vi "Controller Orbit Correction Algorithm.vi"(0 "FOFB Variables":T1, 1 "Corrector Kick Vector in":dbl[](array[numeric]), 2 "Beam Position Vector":dbl[](array[numeric]), 5 "error in (no error)":errorcluster, 9 "Reset?":bool) -> (14 "Good value?":bool=TRUE, 15 "Corrector Kick Vector out":dbl[](array[numeric]), 19 "error out":errorcluster)   [LabVIEW 2011, in "Controller VIs.lvlib"]
doc: "Computes the correction algorithm to the selected BPM readings and returns the calculated corrector kick vector to be applied to the FOFB actuators."
uses:
  Controller VIs.lvlib
  Types Definitions/Type FOFB Variables.ctl
  Common VIs.lvlib
  Type Definitions.lvlib
panel:
  in  "Maximum allowed disturbance (mm) (1.5)":dbl=1.5 format="%#_6f"
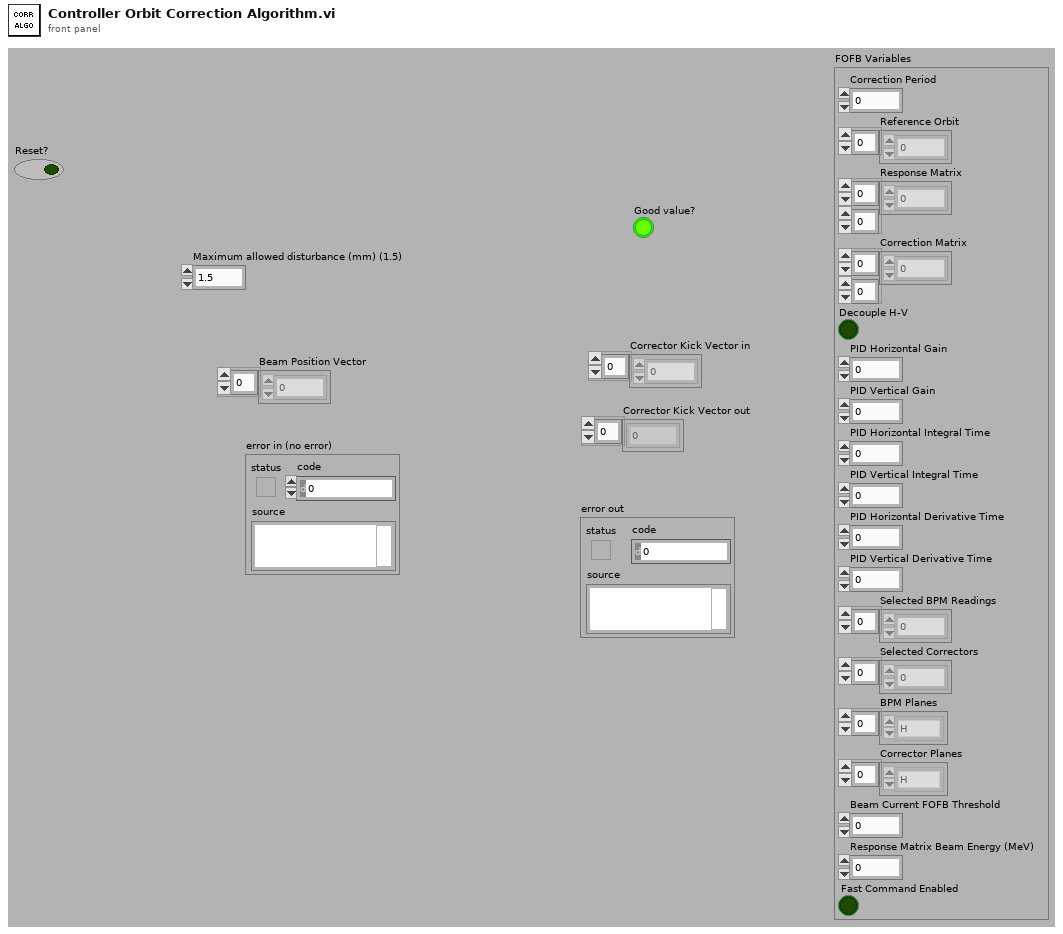
[diagram p1: front panel]
types:
  T1 = typedef "Type Definitions.lvlib/Type FOFB Variables.ctl" = cluster{"Correction Period":u32, "Reference Orbit":dbl[], "Response Matrix":dbl[][], "Correction Matrix":dbl[][], "Decouple H-V":bool, "PID Horizontal Gain":dbl, "PID Vertical Gain":dbl, "PID Horizontal Integral Time":dbl, "PID Vertical Integral Time":dbl, "PID Horizontal Derivative Time":dbl, "PID Vertical Derivative Time":dbl, "Selected BPM Readings":u32[], "Selected Correctors":u32[], "BPM Planes":enum8{"H", "V"}[], "Corrector Planes":enum8{"H", "V"}[], "Beam Current FOFB Threshold":dbl, "Response Matrix Beam Energy (MeV)":dbl, "Fast Command Enabled":bool}
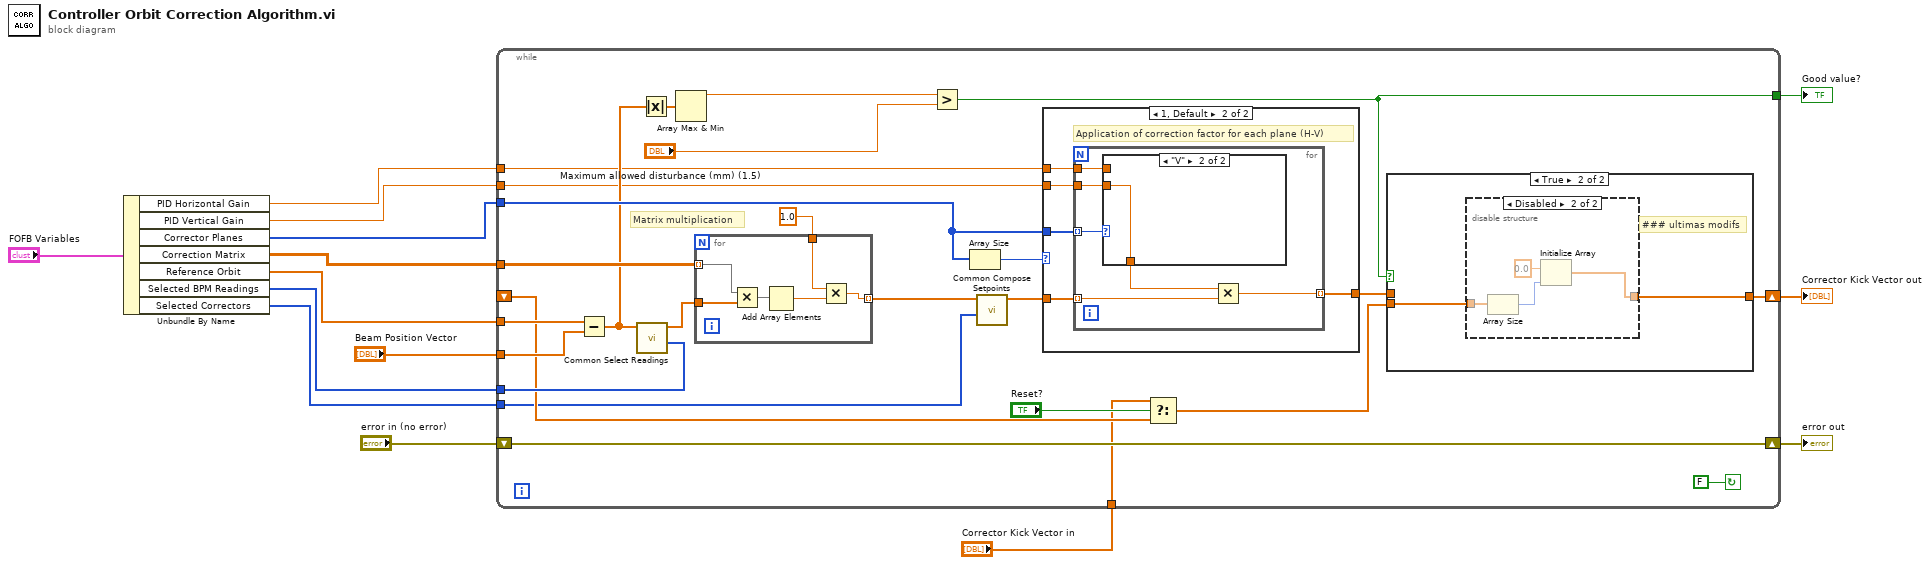
[diagram p0: block diagram]
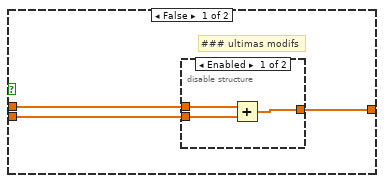
[diagram p2: hidden frame]
diagram:
  n1 = Unbundle By Name("FOFB Variables") -> ("PID Horizontal Gain"=w1:dbl, "PID Vertical Gain"=w2:dbl, "Corrector Planes"=w3:enum8{"H", "V"}[], "Correction Matrix"=w5:dbl[][], "Reference Orbit"=w10:dbl[], "Selected BPM Readings"=w7:u32[], "Selected Correctors"=w6:u32[])
  n2 = while {
    tunnel: w5 -> [w40]
    tunnel: w10 -> [w38]
    tunnel: "Beam Position Vector" -> [w37]
    shift-right: [w36] -> w12
    shift-left: "error in (no error)" -> [w36]
    shift-right: [w31] -> w14
    shift-left: _ -> [w30]
    tunnel: w3 -> [w34]
    tunnel: w7 -> [w33]
    tunnel: w6 -> [w19]
    tunnel: w1 -> [w22]
    tunnel: w2 -> [w21]
    tunnel: [w18] -> w9
    tunnel: "Corrector Kick Vector in" -> [w17]
    stop <- FALSE continue-if-true
    # "Matrix multiplication"
    n3 = Subtract(x=w38, y=w37) -> (x-y=w25:dbl[])
    n4 = call "Common Select Readings.vi"("Selected Readings"=w33, "Readings"=w25) -> ("Readings Subset"=w27:dbl[])  [unwired: 9 in]
    n5 = Absolute Value(x=w25) -> (abs(x)=w24:dbl[])
    n6 = Array Max & Min(array=w24) -> (max value=w16:dbl)  [unwired: 3 out]
    n7 = for {
      tunnel: w27 -> [w60]
      tunnel: w40 -> [w59] mode=indexing
      tunnel: [w56] -> w28 mode=indexing
      tunnel: 1.0 -> [w55]
      n8 = Multiply(x=w59, y=w60) -> (x*y=w58:dbl[])
      n9 = Add Array Elements(numeric array=w58) -> (sum=w57:dbl)
      n10 = Multiply(x=w55, y=w57) -> (x*y=w56:dbl)
    }
    n11 = Greater?(x=w16, y="Maximum allowed disturbance (mm) (1.5)") -> (0:w18:bool)
    n12 = Array Size(array=w34) -> (size(s)=w35:i32)
    n13 = call "Common Compose Setpoints.vi"("Selected Correctors"=w19, "Corrector Kicks Subset"=w28) -> ("Corrector Kicks"=w26:dbl[])  [unwired: 9 in]
    n14 = case shown="1, Default" w35 {
      tunnel: w26 -> [w61 w66]
      tunnel: [w61 w65] -> w32
      tunnel: w34 -> [_ w64]
      tunnel: w22 -> [_ w63]
      tunnel: w21 -> [_ w62]
      frame 0 {
      }
      frame 1, Default {
        # "Application of correction factor for each plane (H-V)"
        n15 = for {
          tunnel: w66 -> [w71] mode=indexing
          tunnel: [w72] -> w65 mode=indexing
          tunnel: w64 -> [w70] mode=indexing
          tunnel: w63 -> [w68]
          tunnel: w62 -> [w67]
          n16 = case shown="\"V\"" w70 {
            tunnel: [w73 w74] -> w69
            tunnel: w68 -> [w73 _]
            tunnel: w67 -> [_ w74]
            frame "H", Default {
            }
            frame "V" {
            }
          }
          n17 = Multiply(x=w69, y=w71) -> (x*y=w72:dbl)
        }
      }
    }
    n18 = Select(t=w17, s="Reset?", f=w30) -> (s? t:f=w29:dbl[])
    n19 = case shown="True" w18 {
      tunnel: w32 -> [w42 _]
      tunnel: [w41 w49] -> w31
      tunnel: w29 -> [w43 w48]
      frame False {
        # "### ultimas modifs"
        n20 = disable-structure shown="Enabled" {
          disable-tunnel: w43 -> [w46 _]
          disable-tunnel: w42 -> [w45 w47]
          disable-tunnel: [w44 w47] -> w41
          frame Enabled {
            n21 = Add(x=w45, y=w46) -> (x+y=w44:dbl[])
          }
          frame Disabled {
          }
        }
      }
      frame True {
        # "### ultimas modifs"
        n22 = disable-structure shown="Disabled" {
          disable-tunnel: [w50 w54] -> w49
          disable-tunnel: w48 -> [w50 w52]
          frame Enabled {
          }
          frame Disabled {
            n23 = Array Size(array=w52) -> (size(s)=w51:i32)
            n24 = Initialize Array(0.0 ("element"), w51) -> (w54:dbl[])
          }
        }
      }
    }
  }
  "error out" <- w12
  "Corrector Kick Vector out" <- w14
  "Good value?" <- w9
